vi "stop.vi"(1 "error in (no error)":errorcluster) -> (0 "error out":errorcluster)   [LabVIEW 2016]
uses:
  sa commands.ctl
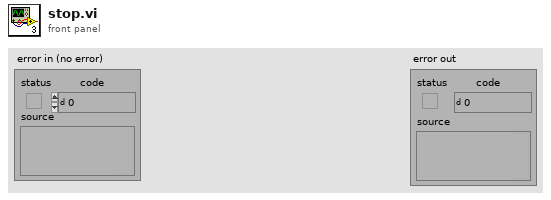
[diagram p1: front panel]
types:
  T1 = typedef "sa commands.ctl" = enum16{"read all", "set system index", "set x channel", "set y channel", "set rotation channel"}
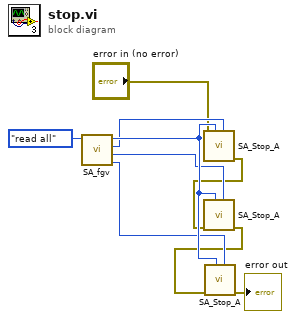
[diagram p0: block diagram]
diagram:
  n1 = call "SA_fgv.vi"("command"=sa_commands."read all") -> ("rotation channel"=w7:u32, "y channel"=w6:u32, "x channel"=w5:u32, "system index"=w8:u32)  [unwired: 3 in]
  n2 = call <vilib>:"SA_Stop_A.vi"("channelIndex"=w5, "systemIndex"=w8, "error in (no error)"="error in (no error)") -> ("error out"=w4:errorcluster)  [unwired: 8 in]
  n3 = call <vilib>:"SA_Stop_A.vi"("channelIndex"=w6, "systemIndex"=w8, "error in (no error)"=w4) -> ("error out"=w3:errorcluster)  [unwired: 8 in]
  n4 = call <vilib>:"SA_Stop_A.vi"("channelIndex"=w7, "systemIndex"=w8, "error in (no error)"=w3) -> ("error out"=→"error out":errorcluster)  [unwired: 8 in]
